vi "Traverse Terminal Data To Source.vi"(0 "Terminal in":refnum<vi>, 5 "Node Tests":refnum<class "Node Test.lvclass">[](array[class]), 11 "error in (no error)":errorcluster) -> (4 "Source Terminals":refnum<vi>[](array[refnum]), 15 "error out":errorcluster)   [LabVIEW 2019, in "MVA Message Mapper.lvlib"]
uses:
  MVA Message Mapper.lvlib
  support/Traversal Algorithm/Node Test.lvclass
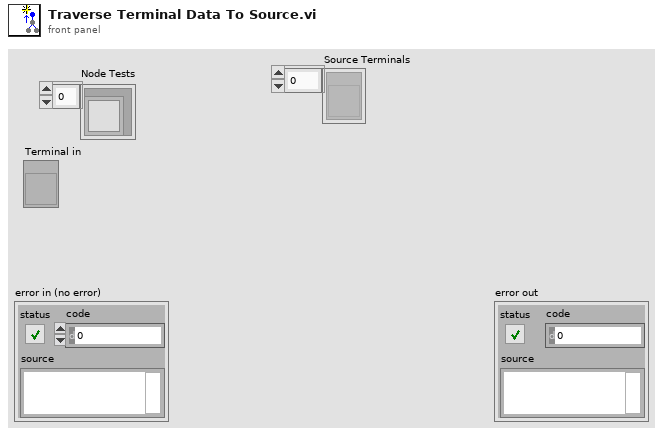
[diagram p1: front panel]
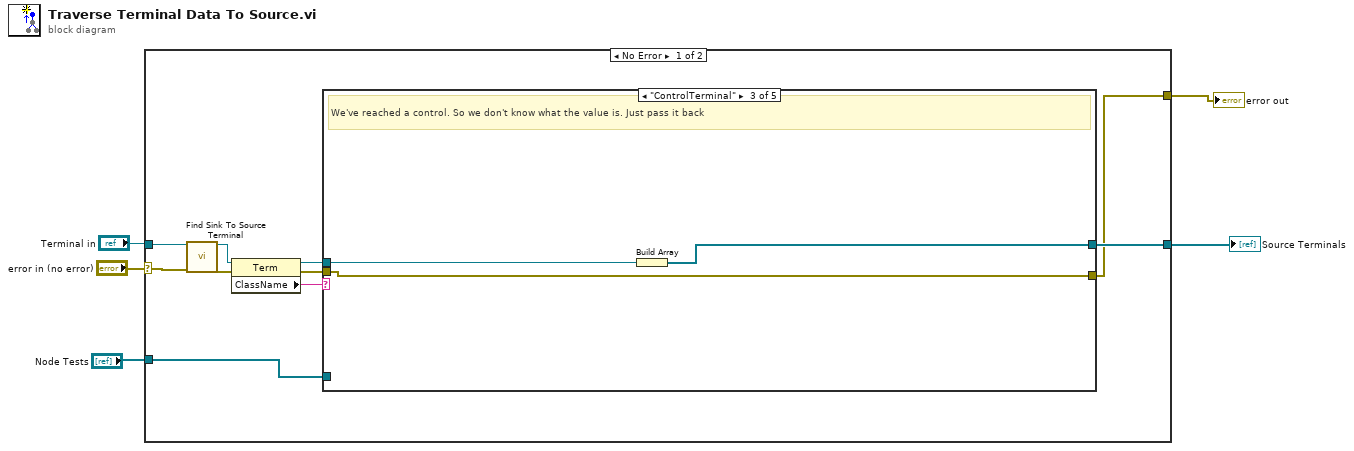
[diagram p0: block diagram]
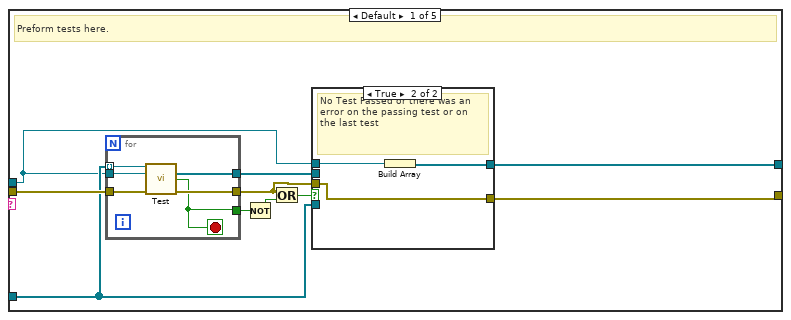
[diagram p2: hidden frame]
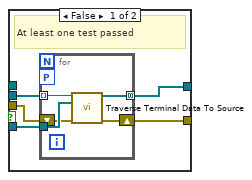
[diagram p3: hidden frame]
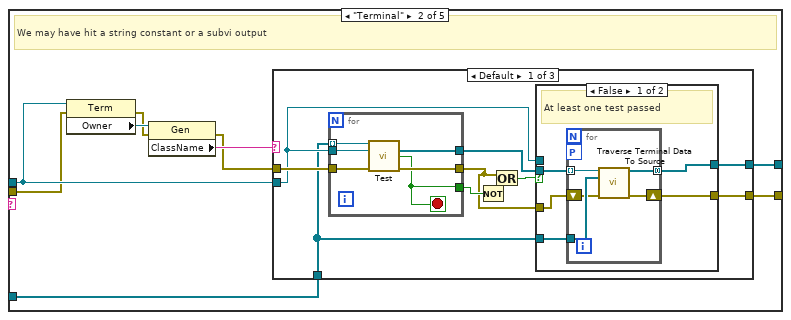
[diagram p4: hidden frame]
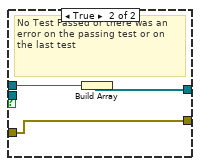
[diagram p5: hidden frame]
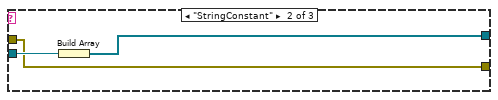
[diagram p6: hidden frame]
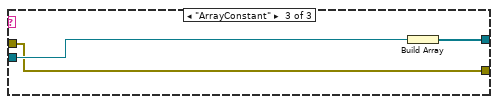
[diagram p7: hidden frame]
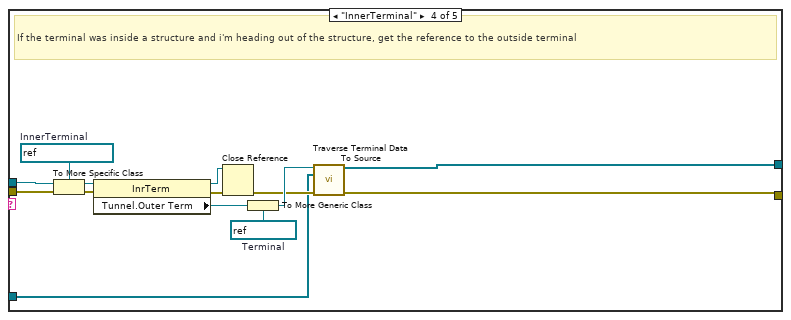
[diagram p8: hidden frame]
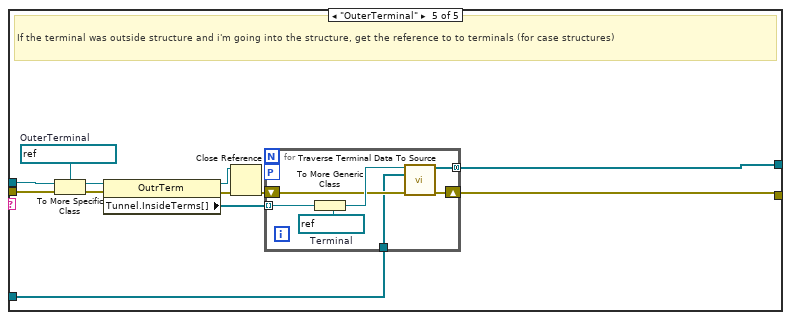
[diagram p9: hidden frame]
diagram:
  n1 = case shown="No Error" "error in (no error)" {
    selector: "error in (no error)" -> [w15 w125]
    tunnel: "Terminal in" -> [w8 _]
    tunnel: [w7 w125] -> w4
    tunnel: "Node Tests" -> [w14 _]
    tunnel: [w13 _] -> w2
    frame No Error {
      n2 = call "Find Sink To Source Terminal.vi"("Source Terminal"=w8, "error in (no error)"=w15) -> ("Sink Terminal"=w6:refnum<vi>, "error out"=w9:errorcluster)  [unwired: 12 in]
      n3 = property class="Term"(reference=w6, error in=w9) -> (reference out=w10:refnum<vi>, error out=w11:errorcluster, "ClassName"=w12:string)
      n4 = case shown="\"ControlTerminal\"" w12 {
        tunnel: w10 -> [w18 w52 w89 w105 w114]
        tunnel: [w25 w53 w91 w98 w112] -> w13
        tunnel: w11 -> [w24 w47 w90 w97 w111]
        tunnel: w14 -> [w22 w49 _ w93 w107]
        tunnel: [w16 w45 w90 w92 w106] -> w7
        frame Default {
          # "Preform tests here."
          n5 = for {
            tunnel: w22 -> [w44] mode=indexing
            tunnel: w18 -> [w43]
            tunnel: w24 -> [w42]
            tunnel: [w41] -> w17
            tunnel: [w40] -> w23
            tunnel: [w39] -> w20
            stop <- w39 stop-if-true
            n6 = call-dynamic "Test.vi"("Traverse Algorithm in"=w44, "Terminal To Identify"=w43, "error in (no error)"=w42) -> ("Terminal for Traversal Continuation"=w40:refnum<vi>[], "Node Identified"=w39:bool, "error out"=w41:errorcluster)  [unwired: 9 in, 1 out]
          }
          n7 = Not(x=w20) -> (.not. x?=w19:bool)
          n8 = Or(x=w17, y=w19) -> (x .or. y?=w21:bool)
          n9 = case shown="True" w21 {
            tunnel: [w30 w37] -> w25
            tunnel: w23 -> [w29 _]
            tunnel: w22 -> [w28 _]
            tunnel: w18 -> [_ w38]
            tunnel: w17 -> [w27 w36]
            tunnel: [w26 w36] -> w16
            frame False {
              # "At least one test passed"
              n10 = for {
                tunnel: [w35] -> w30 mode=concatenating
                tunnel: w29 -> [w34] mode=indexing
                tunnel: w28 -> [w33]
                workers-P: _ -> [_]
                shift-right: [w31] -> w26
                shift-left: w27 -> [w32]
                n11 = call "Traverse Terminal Data To Source.vi"("Terminal in"=w34, "Node Tests"=w33, "error in (no error)"=w32) -> ("Source Terminals"=w35:refnum<vi>[], "error out"=w31:errorcluster)  [unwired: 11 in]
              }
            }
            frame True {
              # "No Test Passed or there was an error on the passing test or on the last test"
              n12 = Build Array(w38) -> (w37:refnum<vi>[])
            }
          }
        }
        frame "Terminal" {
          # "We may have hit a string constant or a subvi output"
          n13 = property class="Term"(reference=w52, error in=w47) -> (error out=w46:errorcluster, "Owner"=w51:refnum<vi>)  [unwired: 1 out]
          n14 = property class="Gen"(reference=w51, error in=w46) -> (error out=w48:errorcluster, "ClassName"=w50:string)  [unwired: 1 out]
          n15 = case shown="Default" w50 {
            tunnel: [w56 w85 w88] -> w53
            tunnel: w52 -> [w61 w84 w87]
            tunnel: w49 -> [w57 _ _]
            tunnel: w48 -> [w63 w83 w86]
            tunnel: [w54 w83 w86] -> w45
            frame Default {
              n16 = for {
                tunnel: w57 -> [w82] mode=indexing
                tunnel: w61 -> [w81]
                tunnel: [w80] -> w55
                tunnel: [w79] -> w62
                tunnel: [w78] -> w59
                tunnel: w63 -> [w77]
                stop <- w78 stop-if-true
                n17 = call-dynamic "Test.vi"("Traverse Algorithm in"=w82, "Terminal To Identify"=w81, "error in (no error)"=w77) -> ("Terminal for Traversal Continuation"=w79:refnum<vi>[], "Node Identified"=w78:bool, "error out"=w80:errorcluster)  [unwired: 9 in, 1 out]
              }
              n18 = Not(x=w59) -> (.not. x?=w60:bool)
              n19 = Or(x=w55, y=w60) -> (x .or. y?=w58:bool)
              n20 = case shown="False" w58 {
                tunnel: [w68 w75] -> w56
                tunnel: w62 -> [w67 _]
                tunnel: w57 -> [w66 _]
                tunnel: w61 -> [_ w76]
                tunnel: w55 -> [w65 w74]
                tunnel: [w64 w74] -> w54
                frame False {
                  # "At least one test passed"
                  n21 = for {
                    tunnel: [w73] -> w68 mode=concatenating
                    tunnel: w67 -> [w72] mode=indexing
                    tunnel: w66 -> [w71]
                    workers-P: _ -> [_]
                    shift-right: [w69] -> w64
                    shift-left: w65 -> [w70]
                    n22 = call "Traverse Terminal Data To Source.vi"("Terminal in"=w72, "Node Tests"=w71, "error in (no error)"=w70) -> ("Source Terminals"=w73:refnum<vi>[], "error out"=w69:errorcluster)  [unwired: 11 in]
                  }
                }
                frame True {
                  # "No Test Passed or there was an error on the passing test or on the last test"
                  n23 = Build Array(w76) -> (w75:refnum<vi>[])
                }
              }
            }
            frame "StringConstant" {
              n24 = Build Array(w84) -> (w85:refnum<vi>[])
            }
            frame "ArrayConstant" {
              n25 = Build Array(w87) -> (w88:refnum<vi>[])
            }
          }
        }
        frame "ControlTerminal" {
          # "We've reached a control. So we don't know what the value is. Just pass it back"
          n26 = Build Array(w89) -> (w91:refnum<vi>[])
        }
        frame "InnerTerminal" {
          w101 = refnum<vi> refnum  # Terminal
          w104 = refnum<vi> refnum  # InnerTerminal
          # "If the terminal was inside a structure and i'm heading out of the structure, get the reference to the outside terminal"
          n27 = To More Specific Class(target class=w104, reference=w105, error in=w97) -> (specific class reference=w103:refnum<vi>, error out=w96:errorcluster)
          n28 = property class="InrTerm"(reference=w103, error in=w96) -> (reference out=w100:refnum<vi>, error out=w95:errorcluster, "Tunnel.Outer Term"=w102:refnum<vi>)
          n29 = Close Reference(reference=w100, error in (no error)=w95) -> (error out=w94:errorcluster)
          n30 = To More Generic Class(target class=w101, reference=w102) -> (generic class reference=w99:refnum<vi>)
          n31 = call "Traverse Terminal Data To Source.vi"("Terminal in"=w99, "Node Tests"=w93, "error in (no error)"=w94) -> ("Source Terminals"=w98:refnum<vi>[], "error out"=w92:errorcluster)  [unwired: 11 in]
        }
        frame "OuterTerminal" {
          w117 = refnum<vi> refnum  # OuterTerminal
          # "If the terminal was outside structure and i'm going into the structure, get the reference to to terminals (for case structures)"
          n32 = To More Specific Class(target class=w117, reference=w114, error in=w111) -> (specific class reference=w116:refnum<vi>, error out=w110:errorcluster)
          n33 = property class="OutrTerm"(reference=w116, error in=w110) -> (reference out=w115:refnum<vi>, error out=w109:errorcluster, "Tunnel.InsideTerms[]"=w113:refnum<vi>[])
          n34 = Close Reference(reference=w115, error in (no error)=w109) -> (error out=w108:errorcluster)
          n35 = for {
            tunnel: w113 -> [w123] mode=indexing
            tunnel: [w121] -> w112 mode=concatenating
            tunnel: w107 -> [w119]
            workers-P: _ -> [_]
            shift-right: [w118] -> w106
            shift-left: w108 -> [w120]
            w124 = refnum<vi> refnum  # Terminal
            n36 = To More Generic Class(target class=w124, reference=w123) -> (generic class reference=w122:refnum<vi>)
            n37 = call "Traverse Terminal Data To Source.vi"("Terminal in"=w122, "Node Tests"=w119, "error in (no error)"=w120) -> ("Source Terminals"=w121:refnum<vi>[], "error out"=w118:errorcluster)  [unwired: 11 in]
          }
        }
      }
    }
    frame Error {
    }
  }
  "error out" <- w4
  "Source Terminals" <- w2
